vi "2 Ball Double Hot Half v2.vi"(1 "Run?":bool) -> (0 "Done?":bool)   [LabVIEW 2013]
uses:
  Globals/Homes.vi
  Globals/Useful Values.vi
panel:
  out "Time Elapsed":dbl
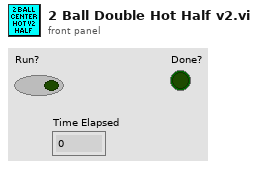
[diagram p1: front panel]
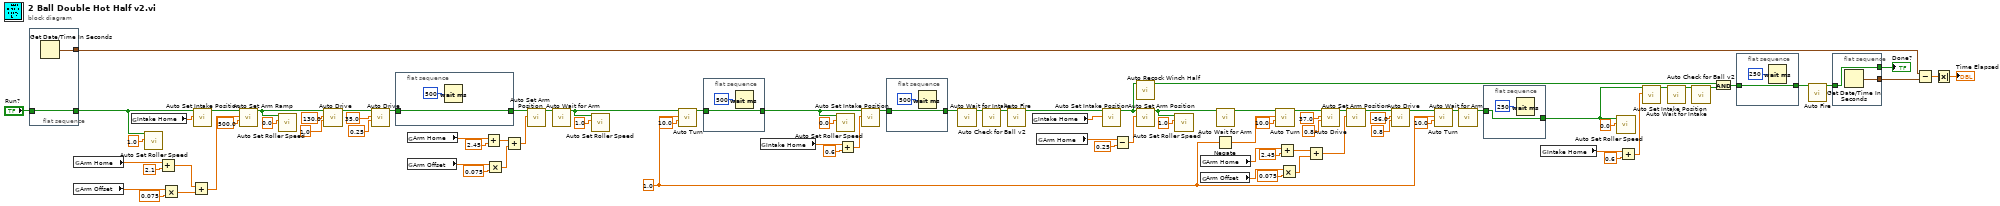
[diagram p0: block diagram]
diagram:
  w7 = 1.0 ("+/-?")
  n1 = flat-sequence {
    tunnel: "Run?" -> [w92]
    tunnel: [w92] -> w10
    tunnel: [w91] -> w46
    frame #0 {
      n2 = Get Date/Time In Seconds() -> (seconds since 1Jan1904=w91:timestamp)
    }
  }
  n3 = global read "Homes.vi" "Arm Home"() -> (w89:dbl)
  n4 = global read "Useful Values.vi" "Arm Offset"() -> (w85:dbl)
  n5 = global read "Homes.vi" "Intake Home"() -> (w88:dbl)
  n6 = call "Auto Set Roller Speed.vi"("Value"=1.0, "Run?"=w10) -> ()  [unwired: 9 in, 1 out]
  n7 = Add(x=w89, y=2.1) -> (x+y=w84:dbl)
  n8 = Multiply(x=w85, y=0.075) -> (x*y=w87:dbl)
  n9 = Add(x=w84, y=w87) -> (x+y=w82:dbl)
  n10 = call "Auto Set Intake Position.vi"("Intake Position"=w88, "Run?"=w10) -> ("Done"=w80:bool)  [unwired: 9 in]
  n11 = call "Auto Set Arm Ramp.vi"("Time (ms)"=500.0, "Arm Position"=w82, "Run?"=w80) -> ("Done"=w11:bool)  [unwired: 8 in]
  n12 = call "Auto Set Roller Speed.vi"("Value"=0.0, "Run?"=w11) -> ()  [unwired: 9 in, 1 out]
  n13 = call "Auto Drive.vi"("Speed"=1.0, "Amount"=130.0, "Run?"=w11) -> ("Done"=w21:bool)  [unwired: 8 in]
  n14 = call "Auto Drive.vi"("Speed"=0.25, "Amount"=35.0, "Run?"=w21) -> ("Done"=w22:bool)  [unwired: 8 in]
  n15 = flat-sequence {
    tunnel: w22 -> [w93]
    tunnel: [w93] -> w64
    frame #0 {
      n16 = Wait (ms)(milliseconds to wait=u32 500) -> ()  [unwired: 1 out]
    }
  }
  n17 = global read "Homes.vi" "Arm Home"() -> (w72:dbl)
  n18 = global read "Useful Values.vi" "Arm Offset"() -> (w77:dbl)
  n19 = Add(x=w72, y=2.45) -> (x+y=w78:dbl)
  n20 = Multiply(x=w77, y=0.075) -> (x*y=w75:dbl)
  n21 = Add(x=w78, y=w75) -> (x+y=w73:dbl)
  n22 = call "Auto Set Arm Position.vi"("Arm Position"=w73, "Run?"=w64) -> ("Done"=w71:bool)  [unwired: 9 in]
  n23 = call "Auto Wait for Arm.vi"("Run?"=w71) -> ("Done"=w1:bool)  [unwired: 10 in]
  n24 = call "Auto Set Roller Speed.vi"("Value"=1.0, "Run?"=w1) -> ()  [unwired: 9 in, 1 out]
  n25 = call "Auto Turn.vi"("Turn Amount"=10.0 ("+/-?"), "+/-?"=w7, "Run?"=w1) -> ("Done"=w25:bool)  [unwired: 8 in]
  n26 = flat-sequence {
    tunnel: [w95] -> w12
    tunnel: w25 -> [w95]
    frame #0 {
      n27 = Wait (ms)(milliseconds to wait=u32 500) -> ()  [unwired: 1 out]
    }
  }
  n28 = global read "Homes.vi" "Intake Home"() -> (w42:dbl)
  n29 = call "Auto Set Roller Speed.vi"("Value"=0.0, "Run?"=w12) -> ()  [unwired: 9 in, 1 out]
  n30 = Add(x=w42, y=0.6) -> (x+y=w40:dbl)
  n31 = call "Auto Set Intake Position.vi"("Intake Position"=w40, "Run?"=w12) -> ("Done"=w27:bool)  [unwired: 9 in]
  n32 = flat-sequence {
    tunnel: [w97] -> w28
    tunnel: w27 -> [w97]
    frame #0 {
      n33 = Wait (ms)(milliseconds to wait=u32 500) -> ()  [unwired: 1 out]
    }
  }
  n34 = call "Auto Wait for Intake.vi"("Run?"=w28) -> ("Done"=w35:bool)  [unwired: 10 in]
  n35 = call "Auto Check for Ball v2.vi"("Run?"=w35) -> ("Done"=w63:bool)  [unwired: 10 in]
  n36 = call "Auto Fire.vi"("Run?"=w63) -> ("Done"=w33:bool)  [unwired: 10 in]
  n37 = global read "Homes.vi" "Intake Home"() -> (w31:dbl)
  n38 = global read "Homes.vi" "Arm Home"() -> (w62:dbl)
  n39 = call "Auto Set Intake Position.vi"("Intake Position"=w31, "Run?"=w33) -> ("Done"=w32:bool)  [unwired: 9 in]
  n40 = Subtract(x=w62, y=0.25) -> (x-y=w60:dbl)
  n41 = call "Auto Recock Winch Half.vi"("Run?"=w32) -> ("Done"=w50:bool)  [unwired: 10 in]
  n42 = call "Auto Set Arm Position.vi"("Arm Position"=w60, "Run?"=w32) -> ("Done"=w13:bool)  [unwired: 9 in]
  n43 = call "Auto Set Roller Speed.vi"("Value"=1.0, "Run?"=w13) -> ()  [unwired: 9 in, 1 out]
  n44 = global read "Homes.vi" "Arm Home"() -> (w58:dbl)
  n45 = global read "Useful Values.vi" "Arm Offset"() -> (w54:dbl)
  n46 = Negate(x=w7) -> (-x=w43:dbl)
  n47 = call "Auto Wait for Arm.vi"("Run?"=w13) -> ("Done"=w24:bool)  [unwired: 10 in]
  n48 = call "Auto Turn.vi"("Turn Amount"=10.0, "+/-?"=w43, "Run?"=w24) -> ("Done"=w15:bool)  [unwired: 8 in]
  n49 = Add(x=w58, y=2.45) -> (x+y=w53:dbl)
  n50 = Multiply(x=w54, y=0.075) -> (x*y=w56:dbl)
  n51 = Add(x=w53, y=w56) -> (x+y=w52:dbl)
  n52 = call "Auto Drive.vi"("Speed"=0.8, "Amount"=37.0, "Run?"=w15) -> ("Done"=w26:bool)  [unwired: 8 in]
  n53 = call "Auto Set Arm Position.vi"("Arm Position"=w52, "Run?"=w26) -> ("Done"=w17:bool)  [unwired: 9 in]
  n54 = call "Auto Drive.vi"("Speed"=0.8, "Amount"=-56.0, "Run?"=w17) -> ("Done"=w16:bool)  [unwired: 8 in]
  n55 = call "Auto Turn.vi"("Turn Amount"=10.0, "+/-?"=w7, "Run?"=w16) -> ("Done"=w4:bool)  [unwired: 8 in]
  n56 = call "Auto Wait for Arm.vi"("Run?"=w4) -> ("Done"=w3:bool)  [unwired: 10 in]
  n57 = flat-sequence {
    tunnel: w3 -> [w99]
    tunnel: [w99] -> w2
    frame #0 {
      n58 = Wait (ms)(milliseconds to wait=u32 250) -> ()  [unwired: 1 out]
    }
  }
  n59 = global read "Homes.vi" "Intake Home"() -> (w36:dbl)
  n60 = call "Auto Set Roller Speed.vi"("Value"=0.0, "Run?"=w2) -> ()  [unwired: 9 in, 1 out]
  n61 = Add(x=w36, y=0.6) -> (x+y=w38:dbl)
  n62 = call "Auto Set Intake Position.vi"("Intake Position"=w38, "Run?"=w2) -> ("Done"=w39:bool)  [unwired: 9 in]
  n63 = call "Auto Wait for Intake.vi"("Run?"=w39) -> ("Done"=w34:bool)  [unwired: 10 in]
  n64 = call "Auto Check for Ball v2.vi"("Run?"=w34) -> ("Done"=w51:bool)  [unwired: 10 in]
  n65 = And(x=w50, y=w51) -> (x .and. y?=w6:bool)
  n66 = flat-sequence {
    tunnel: w6 -> [w101]
    tunnel: [w101] -> w5
    frame #0 {
      n67 = Wait (ms)(milliseconds to wait=u32 250) -> ()  [unwired: 1 out]
    }
  }
  n68 = call "Auto Fire.vi"("Run?"=w5) -> ("Done"=w14:bool)  [unwired: 10 in]
  n69 = flat-sequence {
    tunnel: w14 -> [w104]
    tunnel: [w104] -> w48
    tunnel: [w103] -> w47
    frame #0 {
      n70 = Get Date/Time In Seconds() -> (seconds since 1Jan1904=w103:timestamp)
    }
  }
  n71 = Subtract(x=w46, y=w47) -> (x-y=w45:dbl)
  n72 = Absolute Value(x=w45) -> (abs(x)=→"Time Elapsed":dbl)
  "Done?" <- w48
